vi "Gr_resistance_lockin_using_Rgr_probe.vi"() -> ()   [LabVIEW 2024]
uses:
  <vilib>/Analysis/1siggen.llb/Ramp Pattern by Delta.vi
  <vilib>/Utility/file.llb/Write Delimited Spreadsheet (DBL).vi
  <vilib>/Utility/file.llb/Write Delimited Spreadsheet (string).vi
  <vilib>/Analysis/NI_AALBase.lvlib
  <vilib>/Analysis/NI_AALPro.lvlib
  C:/Users/Public/OneDrive/Desktop/Keithley_2450_2470_1_4_0_LV2015_NewReadme2_2450-LV2015-1.4.0/Keithley 2450/Keithley 2450.lvlib
panel:
  out "Rgr vs Vb":cluster{dbl[], dbl[]}(graph)
  in  "Measurement Count":u32=10
  in  "reset?":bool
  in  "save data":string="H:\\My Drive\\Lab\\PPMS\\Measurement\\GaN_1000C_2min_34_56"
  in  "lockin_avgs":i32=10
  out "std voltage measured":dbl format="%0.2f"
  out "mean voltage measured":dbl=6.7979141 format="%0.4f"
  out "std current measured":dbl=1.0038305493714546e-08 format="%0.5e"
  out "mean current measured":dbl=1.7421272433999997e-09 format="%.4e"
  in  "VISA resource name 2450":refnum<visa-resource-name>="GPIB0::1::INSTR"
  in  "Current Limit":dbl=5e-08
  out "Vb":dbl
  in  "loop?":bool=TRUE
  in  "Vb end (V)":dbl format="%#.4f"
  in  "Vb step (V)":dbl format="%#_4f"
  in  "Vb start (V)":dbl format="%#.4f"
  out "R_gr":dbl
  out "Vbox":dbl format="%#_14f"
  in  "lockinwait":u32=50
  out "Vgr":dbl format="%#_14f"
  out "Vref vs Idev":cluster{dbl[], dbl[]}[](graph)
  out "Igr":dbl format="%#_14f"
  in  "Rbox":dbl format="%#_20f"
  out "Sin voltage in":dbl=1.0 format="%#_13f"
  in  "Vmax":dbl format="%.3f"
  in  "Vstep":dbl format="%.5f"
  in  "Vmin":dbl format="%.3f"
  in  "A frequency":dbl=26.7 format="%#_13g"
  in  "B input Connection":u16(ring)=1 items=["Single-Ended Voltage", "Differential Voltage", "1 MOhm Current Gain", "100 MOhm Current Gain"]
  in  "B Reference Source":u8(ring)=1 items=["External", "Internal", "Internal Sweep"]
  in  "B Sensitivity":u16(ring)=26 items=["1 nV/fA", "2 nV/fA", "5 nV/fA", "10 nV/fA", "20 nV/fA", "50 nV/fA", "100 nV/fA", "200 nV/fA", "500 nV/fA", "1 uV/pA", "2 uV/pA", "5 uV/pA", "10 uV/pA", "20 uV/pA", "50 uV/pA", "100 uV/pA", "200 uV/pA", "500 uV/pA", "1 mV/nA", "2 mV/nA", "5 mV/nA", "10 mV/nA", "20 mV/nA", "50 mV/nA", "100 mV/nA", "200 mV/nA", "500 mV/nA", "1 V/uA"]
  in  "LOCKIN1 address":refnum<visa-resource-name>="COM3"
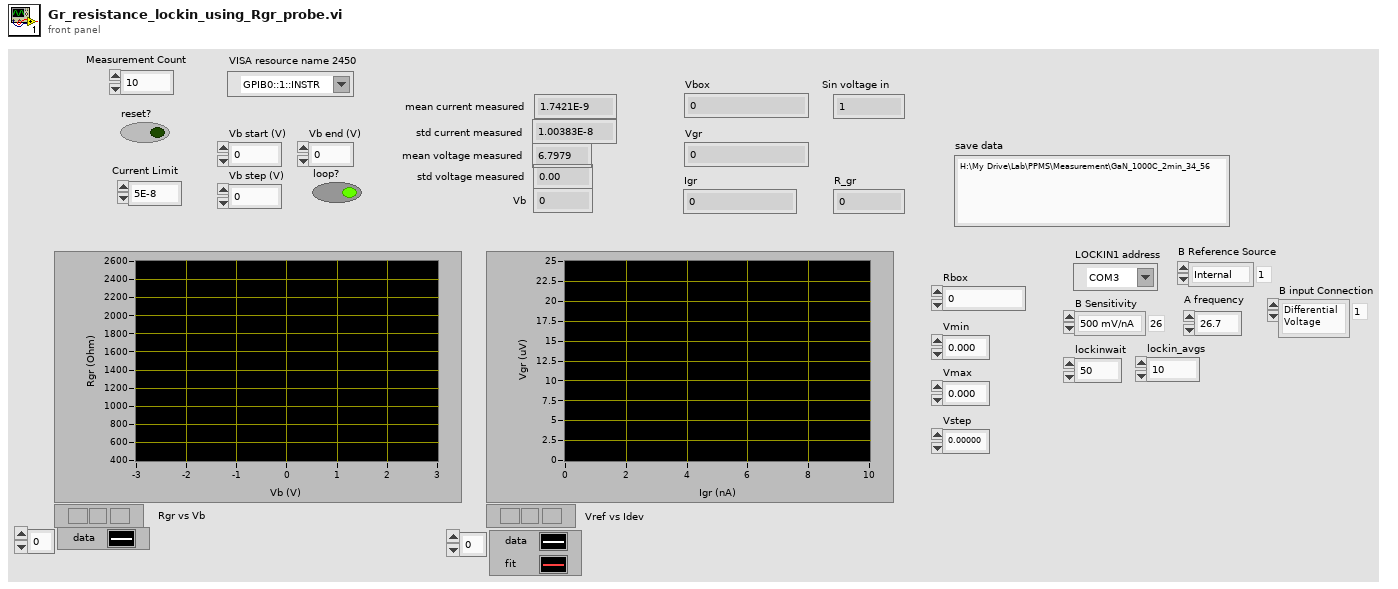
[diagram p1: front panel]
types:
  T1 = enum16{"open", "replace", "create", "open or create", "replace or create", "replace or create with confirmation"}
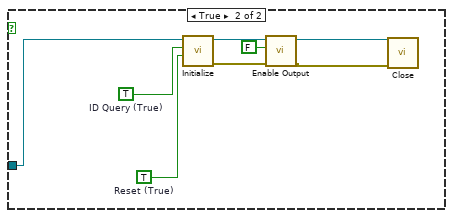
[diagram p3: hidden frame]
diagram:
  w2 = 0
  n1 = Initialize Array(w2, w2) -> (w1:i32[])
  n2 = case shown="False" "reset?" {
    tunnel: "VISA resource name 2450" -> [w9 w462]
    tunnel: w1 -> [w5 _]
    frame False {
      w8 = 0
      w16 = TRUE
      n3 = Negate(x="Vb step (V)") -> (-x=w27:dbl)
      n4 = call-poly <vilib>:"Ramp Pattern.vi"("start"="Vb start (V)", "end"="Vb end (V)", "delta"="Vb step (V)") -> ("samples"=w23:i32, "Ramp Pattern"=w25:dbl[])  [unwired: 6 in, 1 out]
      n5 = call-poly <vilib>:"Ramp Pattern.vi"("start"="Vb end (V)", "end"="Vb start (V)", "delta"=w27) -> ("samples"=w22:i32, "Ramp Pattern"=w24:dbl[])  [unwired: 6 in, 1 out]
      n6 = case shown="True" "loop?" {
        tunnel: w25 -> [w30 w37]
        tunnel: w24 -> [_ w36]
        tunnel: [w30 w32] -> w19
        tunnel: w23 -> [w31 w34]
        tunnel: [w31 w33] -> w20
        tunnel: w22 -> [_ w35]
        frame False {
        }
        frame True {
          n7 = Add(x=w34, y=w35) -> (x+y=w33:i32)
          n8 = Build Array (concatenate)(w37, w36) -> (w32:dbl[])
        }
      }
      n9 = local write "Rbox"("Rbox") -> ()
      n10 = Concatenate Strings("save data", ".txt" ("string")) -> (w11:string)
      n11 = String To Path(string=w11) -> (path=w18:path)
      n12 = call-poly <vilib>:"Write Delimited Spreadsheet.vi"("file path (dialog if empty)"=w18, "append to file? (new file:F)"=w16) -> ("new file path (Not A Path if cancelled)"=w17:path)  [unwired: 12 in, 1 out]
      n13 = Build Array("# Vb_set(V) Vb_meas(V) R_Gr(Ohm) Ib(uA) " ("string")) -> (w14:string[])
      n14 = Initialize Array(w8, w8) -> (w7:i32[])
      n15 = call-poly <vilib>:"Write Delimited Spreadsheet.vi"("file path (dialog if empty)"=w17, "1D data"=w14, "append to file? (new file:F)"=w16) -> ("new file path (Not A Path if cancelled)"=w13:path)  [unwired: 11 in, 1 out]
      n16 = for {
        N: w20 -> [_]
        tunnel: w19 -> [w51] mode=indexing
        tunnel: w9 -> [w73]
        tunnel: w13 -> [w72]
        tunnel: "save data" -> [w71]
        shift-right: [w53] -> _
        shift-left: w7 -> [w62]
        shift-right: [w38] -> _
        shift-left: w5 -> [w47]
        i -> [w52]
        n17 = local write "Vb"(w51) -> ()
        n18 = flat-sequence {
          tunnel: w73 -> [w110]
          tunnel: w62 -> [w104]
          tunnel: [w104] -> w61
          tunnel: w47 -> [w97]
          tunnel: [w97] -> w46
          tunnel: [w212] -> w96
          tunnel: [w211] -> w95
          tunnel: [w207] -> w94
          tunnel: w71 -> [w205]
          tunnel: ["A frequency"] -> w69
          tunnel: [w203] -> w63
          tunnel: w61 -> [w199]
          tunnel: [w199] -> w60
          tunnel: w52 -> [w196]
          tunnel: w46 -> [w193]
          tunnel: [w193] -> w45
          tunnel: w96 -> [w243]
          tunnel: [w243] -> w93
          tunnel: w95 -> [w242]
          tunnel: [w242] -> w92
          tunnel: [w227] -> w91
          tunnel: w94 -> [w241]
          tunnel: ["lockinwait"] -> w74
          tunnel: [w220] -> w70
          tunnel: w69 -> [w220]
          tunnel: [w218] -> w64
          tunnel: w63 -> [w218]
          tunnel: w60 -> [w217]
          tunnel: [w217] -> w59
          tunnel: w45 -> [w214]
          tunnel: [w214] -> w44
          tunnel: [w263] -> w90
          tunnel: [w257] -> w89
          tunnel: w93 -> [w255]
          tunnel: w92 -> [w256]
          tunnel: [w254] -> w88
          tunnel: w91 -> [w254]
          tunnel: w70 -> [w247]
          tunnel: [w246] -> w65
          tunnel: w64 -> [w246]
          tunnel: w59 -> [w245]
          tunnel: [w245] -> w58
          tunnel: w44 -> [w244]
          tunnel: [w244] -> w43
          tunnel: w90 -> [w270]
          tunnel: w89 -> [w271]
          tunnel: [w271] -> w87
          tunnel: [w270] -> w86
          tunnel: [w269] -> w85
          tunnel: w88 -> [w269]
          tunnel: [w267] -> w66
          tunnel: w65 -> [w267]
          tunnel: w58 -> [w266]
          tunnel: [w266] -> w57
          tunnel: w43 -> [w265]
          tunnel: [w265] -> w42
          tunnel: w76 -> [w288]
          tunnel: w75 -> [w287]
          tunnel: w87 -> [w286]
          tunnel: w86 -> [w285]
          tunnel: w85 -> [w284]
          tunnel: [w279] -> w84
          tunnel: [w278] -> w83
          tunnel: [w277] -> w82
          tunnel: w74 -> [w276]
          tunnel: [w275] -> w67
          tunnel: w66 -> [w275]
          tunnel: w57 -> [w274]
          tunnel: [w274] -> w56
          tunnel: [w273] -> w48
          tunnel: w42 -> [w272]
          tunnel: [w272] -> w41
          tunnel: w84 -> [w423]
          tunnel: w83 -> [w422]
          tunnel: w82 -> [w417]
          tunnel: w72 -> [w433]
          tunnel: [w430] -> w68
          tunnel: w67 -> [w430]
          tunnel: w56 -> [w428]
          tunnel: [w427] -> w54
          tunnel: [w423] -> w50
          tunnel: [w422] -> w49
          tunnel: w48 -> [w418]
          tunnel: w41 -> [w421]
          tunnel: [w420] -> w40
          tunnel: [w445] -> w81
          tunnel: [w444] -> w80
          tunnel: w68 -> [w454]
          tunnel: [w438] -> w55
          tunnel: w54 -> [w438]
          tunnel: w50 -> [w447]
          tunnel: w49 -> [w446]
          tunnel: w40 -> [w437]
          tunnel: [w437] -> w39
          tunnel: w81 -> [w461]
          tunnel: w80 -> [w460]
          tunnel: [w459] -> w53
          tunnel: w55 -> [w459]
          tunnel: [w458] -> w38
          tunnel: w39 -> [w458]
          frame #0 {
            n19 = flat-sequence {
              tunnel: w110 -> [w126]
              tunnel: [w120] -> w103
              tunnel: [w119] -> w101
              tunnel: ["Measurement Count"] -> w99
              tunnel: w103 -> [w148]
              tunnel: [w148] -> w102
              tunnel: w101 -> [w147]
              tunnel: [w147] -> w100
              tunnel: w99 -> [w146]
              tunnel: [w146] -> w98
              tunnel: w102 -> [w156]
              tunnel: w100 -> [w155]
              tunnel: [w154] -> w109
              tunnel: [w153] -> w108
              tunnel: w98 -> [w151]
              tunnel: [w151] -> w105
              tunnel: w109 -> [w175]
              tunnel: w108 -> [w174]
              tunnel: [w173] -> w107
              tunnel: [w172] -> w106
              tunnel: w105 -> [w169]
              tunnel: w107 -> [w188]
              tunnel: w106 -> [w189]
              frame #0 {
                w128 = u16 2 items=["Volts", "Current", "Resistance"] ("Function (0: Volts)")
                w135 = u16 0 items=["Voltage", "Current"]  # Source Mode  (0: Voltage)
                w136 = u16 1 items=["Volts", "Current", "Auto Resistance", "Manual Resistance", "Digitize Voltage", "Digitize Current"]  # Measurement Mode
                w127 = TRUE  # Enable Auto Range (T:Enable)
                w137 = u16 1 items=["Volts", "Current", "Resistance"]  # Function (0: Volts)
                w138 = u16 0 items=["Volts", "Current", "Resistance"]  # Function (0: Volts)
                w133 = FALSE  # Reset (True)
                n20 = call "Initialize.vi"("Reset (True)"=w133, "VISA resource name"=w126) -> ("error out"=w112:errorcluster, "VISA resource name out"=w117:refnum<visa-resource-name>)  [unwired: 8 in]
                n21 = call "Clear Buffer.vi"("VISA resource name"=w117, "error in (no error)"=w112) -> ("VISA resource name out"=w116:refnum<visa-resource-name>, "error out"=w113:errorcluster)  [unwired: 12 in]
                n22 = call "Clear Buffer Statistics.vi"("VISA resource name"=w116, "error in (no error)"=w113) -> ("VISA resource name out"=w115:refnum<visa-resource-name>, "error out"=w114:errorcluster)  [unwired: 12 in]
                n23 = call "Configure Measurement Range.vi"("error in (no error)"=w114, "Enable Auto Range (T:Enable)"=w127, "Function (0: Volts)"=w138, "VISA resource name"=w115) -> ("error out"=w140:errorcluster, "VISA resource name out"=w139:refnum<visa-resource-name>)  [unwired: 6 in]
                n24 = call "Configure Measurement Range.vi"("error in (no error)"=w140, "Enable Auto Range (T:Enable)"=w127, "Function (0: Volts)"=w137, "VISA resource name"=w139) -> ("error out"=w131:errorcluster, "VISA resource name out"=w132:refnum<visa-resource-name>)  [unwired: 6 in]
                n25 = local read "Vb"() -> (w111:dbl)
                n26 = call "Configure Measurement Range.vi"("error in (no error)"=w131, "Enable Auto Range (T:Enable)"=w127, "Function (0: Volts)"=w128, "VISA resource name"=w132) -> ("error out"=w130:errorcluster, "VISA resource name out"=w129:refnum<visa-resource-name>)  [unwired: 6 in]
                n27 = call "Configure Output.vi"("VISA resource name"=w129, "Source Level (0)"=w111, "Source Mode  (0: Voltage)"=w135, "Source Limit Level (0.1)"="Current Limit", "error in (no error)"=w130) -> ("VISA resource name out"=w141:refnum<visa-resource-name>, "error out"=w142:errorcluster)  [unwired: 9 in]
                n28 = call "Configure Source Function.vi"("error in (no error)"=w142, "Function (0: Volts)"=w135, "VISA resource name"=w141) -> ("error out"=w143:errorcluster, "VISA resource name out"=w144:refnum<visa-resource-name>)  [unwired: 7 in]
                n29 = call "Configure Measurement Function.vi"("error in (no error)"=w143, "Function (0: Volts)"=w136, "VISA resource name"=w144) -> ("error out"=w124:errorcluster, "VISA resource name out"=w125:refnum<visa-resource-name>)  [unwired: 7 in]
                n30 = call "Set Measurement Count.vi"("error in (no error)"=w124, "Measurement Count"="Measurement Count", "VISA resource name"=w125) -> ("error out"=w122:errorcluster, "VISA resource name out"=w123:refnum<visa-resource-name>)  [unwired: 7 in]
                n31 = call "Enable Output.vi"("error in (no error)"=w122, "Enable Output (T: Enable)"=TRUE, "VISA resource name"=w123) -> ("error out"=w119:errorcluster, "VISA resource name out"=w120:refnum<visa-resource-name>)  [unwired: 7 in]
              }
              frame #1 {
                n32 = Wait (ms)(milliseconds to wait=200) -> ()  [unwired: 1 out]
              }
              frame #2 {
                w157 = 1000000.0 ("Timeout (10000 ms)")
                n33 = call "Make Reading and Store in Buffer.vi"("VISA resource name"=w156, "error in (no error)"=w155) -> ("VISA resource name out"=w165:refnum<visa-resource-name>, "error out"=w166:errorcluster)  [unwired: 12 in]
                n34 = call "Read (Multiple Points).vi"("VISA resource name"=w165, "Start Index (1)"=u32 1, "End Index (1)"=w151, "error in (no error)"=w166) -> ("VISA resource name out"=w154:refnum<visa-resource-name>, "Data out"=w160:string, "error out"=w153:errorcluster)  [unwired: 9 in]
                n35 = Spreadsheet String To Array(delimiter (Tab)=",", format string="%s", spreadsheet string=w160, array type (2D Dbl)=dbl[] []) -> (array=w159:dbl[])
                n36 = call <vilib>:"Std Deviation and Variance.vi"("X"=w159) -> ("mean"=w152:dbl, "standard deviation"=w158:dbl)  [unwired: 1 in, 1 out]
                n37 = Multiply(x=w158, y=w157) -> (x*y=→"std current measured":dbl)
                n38 = Multiply(x=w157, y=w152) -> (x*y=w150:dbl)
                "mean current measured" <- w150
                n39 = local write "mean current measured"(w150) -> ()
              }
              frame #3 {
                n40 = call "Configure Measurement Function.vi"("error in (no error)"=w174, "VISA resource name"=w175) -> ("error out"=w182:errorcluster, "VISA resource name out"=w186:refnum<visa-resource-name>)  [unwired: 8 in]
                n41 = call "Set Measurement Count.vi"("error in (no error)"=w182, "Measurement Count"=w169, "VISA resource name"=w186) -> ("error out"=w183:errorcluster, "VISA resource name out"=w181:refnum<visa-resource-name>)  [unwired: 7 in]
                n42 = Increment(x=w169) -> (x+1=w170:u32)
                n43 = Add(x=w169, y=w169) -> (x+y=w168:u32)
                n44 = call "Make Reading and Store in Buffer.vi"("VISA resource name"=w181, "error in (no error)"=w183) -> ("VISA resource name out"=w185:refnum<visa-resource-name>, "error out"=w184:errorcluster)  [unwired: 12 in]
                n45 = call "Read (Multiple Points).vi"("VISA resource name"=w185, "Start Index (1)"=w170, "End Index (1)"=w168, "error in (no error)"=w184) -> ("VISA resource name out"=w172:refnum<visa-resource-name>, "Data out"=w177:string, "error out"=w173:errorcluster)  [unwired: 9 in]
                n46 = Spreadsheet String To Array(delimiter (Tab)=",", format string="%s", spreadsheet string=w177, array type (2D Dbl)=dbl[] []) -> (array=w176:dbl[])
                n47 = call <vilib>:"Std Deviation and Variance.vi"("X"=w176) -> ("mean"=w167:dbl, "standard deviation"=→"std voltage measured":dbl)  [unwired: 1 in, 1 out]
                "mean voltage measured" <- w167
                n48 = local write "mean voltage measured"(w167) -> ()
              }
              frame #4 {
                n49 = call "Enable Output.vi"("error in (no error)"=w188, "Enable Output (T: Enable)"=TRUE, "VISA resource name"=w189) -> ("error out"=w191:errorcluster, "VISA resource name out"=w192:refnum<visa-resource-name>)  [unwired: 7 in]
                n50 = call "Close.vi"("error in (no error)"=w191, "VISA resource name"=w192) -> ("error out"=w190:errorcluster)  [unwired: 9 in]
                n51 = call <vilib>:"Simple Error Handler.vi"("error in (no error)"=w190) -> ()  [unwired: 4 in, 5 out]
              }
            }
          }
          frame #1 {
            n52 = local read "Vb"() -> (w194:dbl)
            n53 = Multiply(x=w194, y=1000.0) -> (x*y=w202:dbl)
            n54 = Round To Nearest(number=w202) -> (nearest integer value=w201:dbl)
            n55 = Format Into String(format string="%d", w201) -> (resulting string=w209:string)  [unwired: 2 in, 1 out]
            n56 = Format Into String(w196) -> (resulting string=w195:string)  [unwired: 3 in, 1 out]
            n57 = Concatenate Strings(w205, "_VI_data_Vb" ("string"), w209, "mV__" ("string"), w195, "__.txt" ("string")) -> (w203:string)
            n58 = local read "LOCKIN1 address"() -> (w213:refnum<visa-resource-name>)
            n59 = String To Path(string=w203) -> (path=w207:path)
            n60 = Open/Create/Replace File(file path (use dialog)=w207, operation (0:open)=T1."open or create") -> ()  [unwired: 4 in, 3 out]
            n61 = call "OE1022D_OpenDevice.vi"("VISA resource name"=w213) -> ("VISA资源名称输出"=w212:refnum<visa-resource-name>, "错误输出"=w211:errorcluster)  [unwired: 17 in]
          }
          frame #2 {
            w225 = TRUE
            n62 = local read "Rbox"() -> (w216:dbl)
            n63 = local read "Vb"() -> (w215:dbl)
            n64 = Format Into String(initial string="# Rbox (Ohm) = ", w216) -> (resulting string=w240:string)  [unwired: 2 in, 1 out]
            n65 = Format Into String(initial string="# Freq (Hz) = ", w220) -> (resulting string=w219:string)  [unwired: 2 in, 1 out]
            n66 = Build Array(w240) -> (w238:string[])
            n67 = Format Into String(initial string="# Vb(V) = ", w215) -> (resulting string=w226:string)  [unwired: 2 in, 1 out]
            n68 = Format Into String(initial string="# Lockin wait time (ms) = ", "lockinwait") -> (resulting string=w233:string)  [unwired: 2 in, 1 out]
            n69 = Build Array(w226) -> (w222:string[])
            n70 = call-poly <vilib>:"Write Delimited Spreadsheet.vi"("file path (dialog if empty)"=w241, "1D data"=w238, "append to file? (new file:F)"=w225) -> ("new file path (Not A Path if cancelled)"=w237:path)  [unwired: 11 in, 1 out]
            n71 = Build Array(w233) -> (w232:string[])
            n72 = Build Array(w219) -> (w229:string[])
            n73 = Build Array("# Vref(V) Vgr(uV) Igr(nA) Rgr(Ohm) theta(deg)" ("format string")) -> (w223:string[])
            n74 = call-poly <vilib>:"Write Delimited Spreadsheet.vi"("file path (dialog if empty)"=w237, "1D data"=w232, "append to file? (new file:F)"=w225) -> ("new file path (Not A Path if cancelled)"=w235:path)  [unwired: 11 in, 1 out]
            n75 = call-poly <vilib>:"Write Delimited Spreadsheet.vi"("file path (dialog if empty)"=w235, "1D data"=w229, "append to file? (new file:F)"=w225) -> ("new file path (Not A Path if cancelled)"=w230:path)  [unwired: 11 in, 1 out]
            n76 = call-poly <vilib>:"Write Delimited Spreadsheet.vi"("file path (dialog if empty)"=w230, "1D data"=w222, "append to file? (new file:F)"=w225) -> ("new file path (Not A Path if cancelled)"=w228:path)  [unwired: 11 in, 1 out]
            n77 = call-poly <vilib>:"Write Delimited Spreadsheet.vi"("file path (dialog if empty)"=w228, "1D data"=w223, "append to file? (new file:F)"=w225) -> ("new file path (Not A Path if cancelled)"=w227:path)  [unwired: 11 in, 1 out]
          }
          frame #3 {
            w259 = u8 1 items=["Channel A", "Channel B"] ("OE1022D A/B")
            n78 = call "OE1022D_Configure Reference Source.vi"("VISA resource name"=w255, "OE1022D A/B"=w259, "Reference Source"="B Reference Source", "error in (no error)"=w256) -> ("VISA resource name out"=w253:refnum<visa-resource-name>, "error out"=w252:errorcluster)  [unwired: 14 in]
            n79 = call "OE1022D_Configure Frequency.vi"("VISA resource name"=w253, "OE1022D A/B"=w259, "Internal Frequency(Hz)"=w247, "error in (no error)"=w252) -> ("VISA resource name out"=w262:refnum<visa-resource-name>, "error out"=w261:errorcluster)  [unwired: 14 in]
            n80 = call "OE1022D_Configure Ref Phase Channel A.vi"("VISA resource name"=w262, "Reference Source"="B Reference Source", "Internal Frequency(Hz)"=w247, "error in (no error)"=w261) -> ("VISA resource name out"=w248:refnum<visa-resource-name>, "error out"=w249:errorcluster)  [unwired: 14 in]
            n81 = call "OE1022D_Configure Sensitivity.vi"("VISA resource name"=w248, "OE1022D A/B"=w259, "Sensitivity"="B Sensitivity", "error in (no error)"=w249) -> ("VISA resource name out"=w250:refnum<visa-resource-name>, "error out"=w251:errorcluster)  [unwired: 14 in]
            n82 = call "OE1022D_Configure Input Filter.vi"("VISA resource name"=w250, "Input Source"="B input Connection", "OE1022D A/B"=w259, "error in (no error)"=w251) -> ("VISA resource name out"=w257:refnum<visa-resource-name>, "error out"=w263:errorcluster)  [unwired: 10 in]
          }
          frame #4 {
            n83 = Wait (ms)(milliseconds to wait=500) -> ()  [unwired: 1 out]
          }
          frame #5 {
            w281 = 0
            w283 = 0
            n84 = Initialize Array(w283, w283) -> (w282:i32[])
            n85 = Initialize Array(w281, w281) -> (w280:i32[])
            n86 = for {
              N: w288 -> [_]
              tunnel: w287 -> [w291] mode=indexing
              tunnel: w286 -> [w331]
              tunnel: w285 -> [w330]
              tunnel: w284 -> [w329]
              shift-right: [w319] -> w273
              shift-left: w282 -> [w324]
              shift-right: [w311] -> w277
              shift-left: w280 -> [w317]
              tunnel: [w295] -> w278
              tunnel: [w292] -> w279
              tunnel: w276 -> [w297]
              n87 = local write "Sin voltage in"(w291) -> ()
              n88 = flat-sequence {
                tunnel: w331 -> [w338]
                tunnel: w330 -> [w337]
                tunnel: w291 -> [w332]
                tunnel: [w336] -> w310
                tunnel: [w335] -> w308
                tunnel: [w334] -> w306
                tunnel: w324 -> [w334]
                tunnel: w317 -> [w333]
                tunnel: [w333] -> w304
                tunnel: w310 -> [w347]
                tunnel: [w347] -> w309
                tunnel: w308 -> [w346]
                tunnel: [w346] -> w307
                tunnel: w306 -> [w345]
                tunnel: [w345] -> w305
                tunnel: w304 -> [w344]
                tunnel: [w344] -> w303
                tunnel: w297 -> [w343]
                tunnel: w309 -> [w367]
                tunnel: w307 -> [w366]
                tunnel: [w365] -> w327
                tunnel: [w364] -> w326
                tunnel: w305 -> [w369]
                tunnel: [w368] -> w320
                tunnel: w303 -> [w355]
                tunnel: [w354] -> w313
                tunnel: [w362] -> w299
                tunnel: [w374] -> w328
                tunnel: w327 -> [w374]
                tunnel: w326 -> [w373]
                tunnel: [w373] -> w325
                tunnel: [w372] -> w321
                tunnel: w320 -> [w372]
                tunnel: [w371] -> w314
                tunnel: w313 -> [w371]
                tunnel: w299 -> [w370]
                tunnel: [w370] -> w298
                tunnel: w328 -> [w382]
                tunnel: w325 -> [w379]
                tunnel: [w384] -> w322
                tunnel: w321 -> [w384]
                tunnel: [w383] -> w315
                tunnel: w314 -> [w383]
                tunnel: [w380] -> w302
                tunnel: [w381] -> w301
                tunnel: w298 -> [w378]
                tunnel: [w376] -> w289
                tunnel: [w389] -> w323
                tunnel: w322 -> [w389]
                tunnel: [w388] -> w316
                tunnel: w315 -> [w388]
                tunnel: w302 -> [w387]
                tunnel: w301 -> [w386]
                tunnel: [w387] -> w300
                tunnel: [w386] -> w293
                tunnel: [w385] -> w290
                tunnel: w289 -> [w385]
                tunnel: w329 -> [w404]
                tunnel: w323 -> [w401]
                tunnel: [w401] -> w318
                tunnel: w316 -> [w400]
                tunnel: [w400] -> w312
                tunnel: w300 -> [w399]
                tunnel: [w399] -> w296
                tunnel: [w398] -> w294
                tunnel: w293 -> [w398]
                tunnel: w290 -> [w396]
                tunnel: [w407] -> w319
                tunnel: w318 -> [w407]
                tunnel: [w406] -> w311
                tunnel: w312 -> [w406]
                tunnel: [w412] -> w295
                tunnel: w296 -> [w412]
                tunnel: [w411] -> w292
                tunnel: w294 -> [w411]
                frame #0 {
                  n89 = Format Into String(format string="SLVLD2,%.4f;", w332) -> (resulting string=w341:string)  [unwired: 2 in, 1 out]
                  n90 = Concatenate Strings(w341, "\r") -> (w342:string)
                  n91 = VISA Write(VISA resource name=w338, write buffer=w342, error in (no error)=w337) -> (VISA resource name out=w336:refnum<visa-resource-name>, error out=w335:errorcluster)  [unwired: 1 out]
                }
                frame #1 {
                  n92 = Wait (ms)(milliseconds to wait=w343) -> ()  [unwired: 1 out]
                }
                frame #2 {
                  w363 = u16 2 items=["X", "Y", "R", "Theta", "Frequency", "Noise", "Xh1", "Yh1", "Rh1", "Theta h1", "Xh2", "Yh2", "Rh2", "Theta h2"] ("Parameter 2")
                  w362 = 1
                  n93 = call "OE1022D_Read 1 parameter_mean_and_std.vi"("Num Averages"="lockin_avgs", "Parameter 2"=w363, "错误输入（无错误）"=w366, "Channel (0: A)"=w362, "VISA resource name"=w367) -> ("error out"=w365:errorcluster, "Measurement"=w350:dbl, "VISA resource name out"=w364:refnum<visa-resource-name>)  [unwired: 3 in, 1 out]
                  n94 = Multiply(x=1000000.0, y=w350) -> (x*y=w348:dbl)
                  "Vgr" <- w348
                  n95 = local read "Sin voltage in"() -> (w356:dbl)
                  n96 = Build Array (concatenate)(w369, w348) -> (w368:dbl[])
                  n97 = local write "Vgr"(w348) -> ()
                  n98 = Subtract(x=w356, y=w350) -> (x-y=w361:dbl)
                  n99 = local read "Rbox"() -> (w357:dbl)
                  n100 = Multiply(x=w361, y=1.0) -> (x*y=w358:dbl)
                  "Vbox" <- w358
                  n101 = Divide(x=w358, y=w357) -> (x/y=w353:dbl)
                  n102 = Multiply(x=w353, y=1000000000.0) -> (x*y=w351:dbl)
                  "Igr" <- w351
                  n103 = local write "Igr"(w351) -> ()
                  n104 = Build Array (concatenate)(w355, w351) -> (w354:dbl[])
                }
                frame #3 {
                  n105 = Wait (ms)(milliseconds to wait=u32 50) -> ()  [unwired: 1 out]
                }
                frame #4 {
                  w377 = u16 3 items=["X", "Y", "R", "Theta", "Frequency", "Noise", "Xh1", "Yh1", "Rh1", "Theta h1", "Xh2", "Yh2", "Rh2", "Theta h2"] ("Parameter 2")
                  n106 = call "OE1022D_Read 1 parameter_mean_and_std.vi"("Parameter 2"=w377, "错误输入（无错误）"=w382, "Channel (0: A)"=w378, "VISA resource name"=w379) -> ("error out"=w381:errorcluster, "Measurement"=w376:dbl, "VISA resource name out"=w380:refnum<visa-resource-name>)  [unwired: 4 in, 1 out]
                }
                frame #5 {
                  n107 = Wait (ms)(milliseconds to wait=u32 50) -> ()  [unwired: 1 out]
                }
                frame #6 {
                  (unwired) "Vref\nVgr\nIgr\nRgr\nTheta"
                  n108 = local read "Sin voltage in"() -> (w397:dbl)
                  n109 = local read "Vgr"() -> (w394:dbl)
                  n110 = local read "Igr"() -> (w395:dbl)
                  n111 = Divide(x=w394, y=w395) -> (x/y=w393:dbl)
                  n112 = Multiply(x=w393, y=1000.0) -> (x*y=w392:dbl)
                  n113 = Build Array(w397, w394, w395, w392, w396) -> (w405:dbl[])
                  n114 = call-poly <vilib>:"Write Delimited Spreadsheet.vi"("file path (dialog if empty)"=w404, "format (%.3f)"="%.12f", "1D data"=w405, "append to file? (new file:F)"=TRUE) -> ()  [unwired: 10 in, 2 out]
                }
                frame #7 {
                  n115 = Bundle(w406, w407) -> (w409:cluster{dbl[], dbl[]})  [unwired: 1 in]
                  n116 = Bundle(w406, w407) -> (w408:cluster{dbl[], dbl[]})  [unwired: 1 in]
                  n117 = Build Array(w408, w409) -> (w410:cluster{dbl[], dbl[]}[])
                  "Vref vs Idev" <- w410
                  n118 = local write "Vref vs Idev"(w410) -> ()
                }
              }
              "Sin voltage in" <- w291
            }
          }
          frame #6 {
            n119 = local read "mean current measured"() -> (w425:dbl)
            n120 = local read "mean voltage measured"() -> (w424:dbl)
            n121 = local read "Vb"() -> (w426:dbl)
            n122 = Bundle(w417, w418) -> (w435:cluster{dbl[], dbl[]})  [unwired: 1 in]
            n123 = call <vilib>:"Linear Fit.vi"("Y"=w418, "X"=w417) -> ("Best Linear Fit"=w416:dbl[], "slope"=w414:dbl)  [unwired: 9 in, 3 out]
            n124 = Bundle(w417, "Best Linear Fit"=w416) -> (w434:cluster{dbl[], "Best Linear Fit":dbl[]})  [unwired: 1 in]
            n125 = Build Array(w435, w434) -> (w431:cluster{dbl[], "Best Linear Fit":dbl[]}[])
            n126 = Multiply(x=w414, y=1000.0) -> (x*y=w413:dbl)
            "R_gr" <- w413
            n127 = Build Array(w426, w424, w413, w425) -> (w432:dbl[])
            n128 = local read "Vb"() -> (w419:dbl)
            n129 = local write "Vref vs Idev"(w431) -> ()
            n130 = call-poly <vilib>:"Write Delimited Spreadsheet.vi"("file path (dialog if empty)"=w433, "format (%.3f)"="%.12f", "1D data"=w432, "append to file? (new file:F)"=TRUE) -> ()  [unwired: 10 in, 2 out]
            n131 = Build Array (concatenate)(w428, w413) -> (w427:dbl[])
            n132 = Build Array (concatenate)(w421, w419) -> (w420:dbl[])
          }
          frame #7 {
            n133 = Concatenate Strings(w454, "_plot" ("format string")) -> (w452:string)
            n134 = String To Path(string=w452) -> (path=w451:path)
            n135 = Bundle(w437, w438) -> (→"Rgr vs Vb":cluster{dbl[], dbl[]})  [unwired: 1 in]
            n136 = invoke on="Vref vs Idev" class="XYGraph (strict)" method="Export Image"("FileType"=enum32{"BMP", "EPS", "EMF", "PICT"}."BMP" ("File Type"), "Target"=enum32{"File", "Clipboard"}."File", "Path"=w451, "HideGrid"=FALSE ("Hide Grid"), "Overwrite"=TRUE ("Always Overwrite")) -> ()  [unwired: 3 in, 8 out]
            n137 = Format Into String(format string="SLVLD2,%.4f;", 0.001 ("input 1")) -> (resulting string=w443:string)  [unwired: 2 in, 1 out]
            n138 = Concatenate Strings(w443, "\r") -> (w439:string)
            n139 = Wait (ms)(milliseconds to wait=u32 100) -> ()  [unwired: 1 out]
            n140 = VISA Write(VISA resource name=w446, write buffer=w439, error in (no error)=w447) -> (VISA resource name out=w444:refnum<visa-resource-name>, error out=w445:errorcluster)  [unwired: 1 out]
          }
          frame #8 {
            n141 = call "OE1022D_Close.vi"("错误输入（无错误）"=w461, "VISA resource name"=w460) -> ()  [unwired: 1 in, 1 out]
          }
        }
        n142 = call-poly <vilib>:"Ramp Pattern.vi"("start"="Vmin", "end"="Vmax", "delta"="Vstep") -> ("samples"=w76:i32, "Ramp Pattern"=w75:dbl[])  [unwired: 6 in, 1 out]
        "Vb" <- w51
      }
    }
    frame True {
      w468 = TRUE  # Reset (True)
      w469 = TRUE  # ID Query (True)
      n143 = call "Initialize.vi"("Reset (True)"=w468, "ID Query (True)"=w469, "VISA resource name"=w462) -> ("error out"=w467:errorcluster, "VISA resource name out"=w466:refnum<visa-resource-name>)  [unwired: 7 in]
      n144 = call "Enable Output.vi"("error in (no error)"=w467, "Enable Output (T: Enable)"=FALSE, "VISA resource name"=w466) -> ("error out"=w464:errorcluster, "VISA resource name out"=w465:refnum<visa-resource-name>)  [unwired: 7 in]
      n145 = call "Close.vi"("error in (no error)"=w464, "VISA resource name"=w465) -> ()  [unwired: 9 in, 1 out]
    }
  }
